vi "hw7p4_hickey.vi"() -> ()   [LabVIEW 2014]
uses:
  <vilib>/MakerHub/LINX/Private/Type Defs/User Platform.ctl
  <vilib>/MakerHub/LINX/Private/Type Defs/Interface.ctl
  <vilib>/MakerHub/LINX/Public/Peripherals/Analog/Analog Read 1 Chan.vi
  <vilib>/MakerHub/LINX/LMH-LINX.lvlib
panel:
  out "Error Out 3":errorcluster
  in  "stop":bool
  out "Error Out 2":errorcluster
  out "AI Value":dbl
  in  "Analog Channel":u8
  in  "Serial Port":refnum<visa-resource-name>="N/A"
  in  "Interface":T1
  in  "Platform":T2
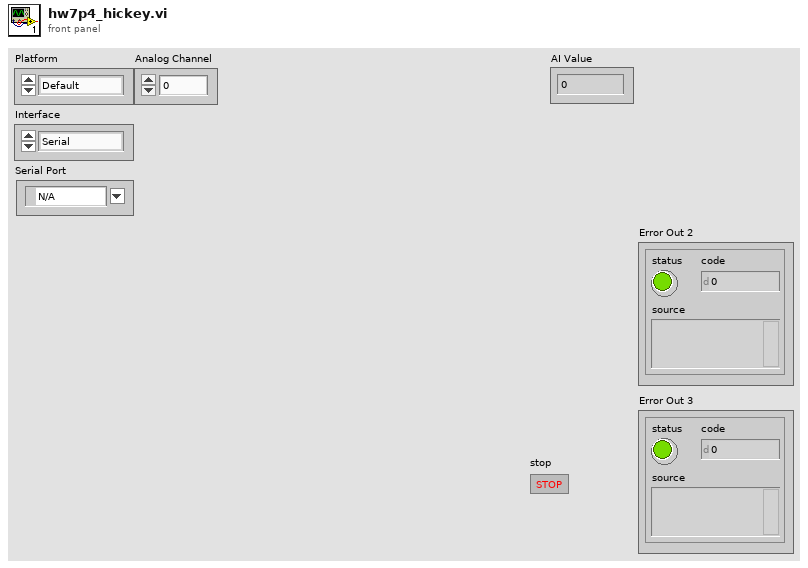
[diagram p1: front panel]
types:
  T1 = typedef "LMH-LINX.lvlib/Interface.ctl" = enum16{"Serial", "TCP"}
  T2 = typedef "LMH-LINX.lvlib/User Platform.ctl" = enum16{"Default", "LINX", "myRIO"}
  T3 = typedef "LMH-LINX.lvlib/LINX Ref.ctl" = cluster{"Platform":T4, "Interface":T1, "LINX Device Config":T5}
  T4 = typedef "LMH-LINX.lvlib/Platform.ctl" = enum16{"LINX", "myRIO"}
  T5 = typedef "LMH-LINX.lvlib/Device.lvlib/LINX Device Config.ctl" = cluster{"Interface":T1, "COM Port":refnum<visa-resource-name>, "TCP Configuration":T6, "Device Family":u8, "Device ID":u8, "Device Name":string, "TCP Ref":refnum<k5>, "Channels":T7}
  T6 = typedef "LMH-LINX.lvlib/Device.lvlib/TCP Config.ctl" = cluster{"IP Address":string, "Port":u16}
  T7 = typedef "LMH-LINX.lvlib/Channels.ctl" = cluster{"DI":u8[], "DO":u8[], "AI":u8[], "AO":u8[], "PWM":u8[], "QE":u8[], "UART":u8[], "I2C 2":u8[], "SPI":u8[], "CAN":u8[], "Servo":u8[], "AI Ref (V)":dbl, "AO Ref (V)":dbl, "AO Resolution (Bits)":u8}
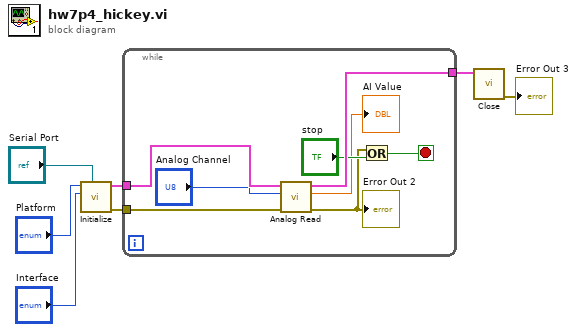
[diagram p0: block diagram]
diagram:
  n1 = call <vilib>:"Initialize.vi"("Serial Port"="Serial Port", "Interface"="Interface", "Platform"="Platform") -> ("Error Out"=w2:errorcluster, "LINX Ref"=w6:T3)  [unwired: 6 in, 1 out]
  n2 = while {
    tunnel: [w15] -> w7
    tunnel: w6 -> [w14]
    tunnel: w2 -> [w13]
    stop <- w10 stop-if-true
    n3 = call-poly <vilib>:"Analog Read.vi"("Error In"=w13, "Analog Channel"="Analog Channel", "LINX Resource"=w14) -> ("Error Out"=w8:errorcluster, "AI Value"=→"AI Value":dbl, "LINX Resource"=w15:T3)  [unwired: 5 in, 1 out]
    "Error Out 2" <- w8
    n4 = Or(x=w8, y="stop") -> (x .or. y?=w10:bool)
  }
  n5 = call <vilib>:"Close.vi"("LINX Resource"=w7) -> ("Error Out"=→"Error Out 3":errorcluster)  [unwired: 9 in, 1 out]
